vi "Configure Trigger (Setup and Hold).vi"(5 "Slope Type (0: Positive)":i32(ring) items=["Positive", "Negative"], 6 "Setup Time (3E-9 S)":dbl=3e-09, 7 "Hold Time (2E-9 S)":dbl=2e-09, 8 "error in (no error)":errorcluster, 9 "Data Source (1: Channel 2)":i32(ring)=1 items=["Channel 1"=0, "Channel 2"=1, "Channel 3"=2, "Channel 4"=3, "D0"=13, "D1"=14, "D2"=15, "D3"=16, "D4"=17, "D5"=18, "D6"=19, "D7"=20, "D8"=21, "D9"=22, "D10"=23, "D11"=24, "D12"=25, "D13"=26, "D14"=27, "D15"=28, "External"=29], 10 "Clock Source (0: Channel 1)":i32(ring) items=["Channel 1"=0, "Channel 2"=1, "Channel 3"=2, "Channel 4"=3, "D0"=13, "D1"=14, "D2"=15, "D3"=16, "D4"=17, "D5"=18, "D6"=19, "D7"=20, "D8"=21, "D9"=22, "D10"=23, "D11"=24, "D12"=25, "D13"=26, "D14"=27, "D15"=28, "External"=29], 11 "VISA resource name":refnum<visa-resource-name>) -> (0 "error out":errorcluster, 3 "VISA resource name out":refnum<visa-resource-name>)   [LabVIEW 2016, in "Agilent 2000 3000 X-Series.lvlib"]
doc: "Configures the setup and hold trigger mode."
uses:
  Agilent 2000 3000 X-Series.lvlib
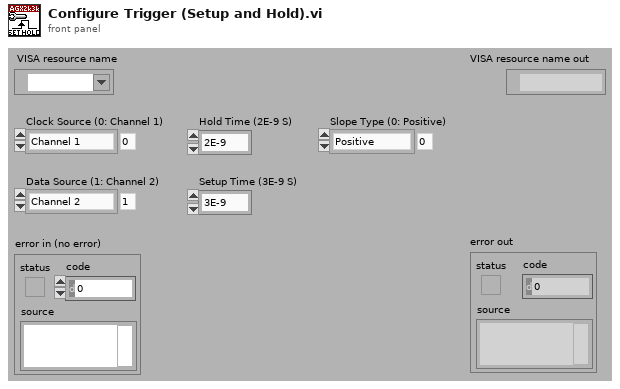
[diagram p1: front panel]
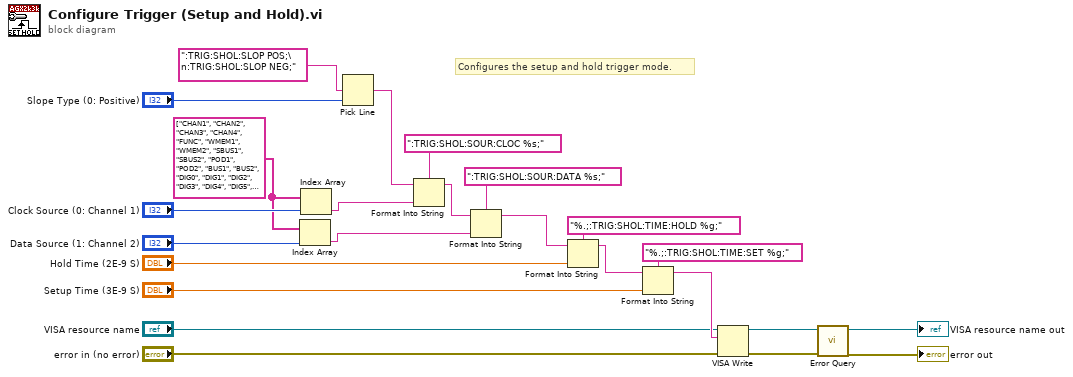
[diagram p0: block diagram]
diagram:
  w3 = string[] ["CHAN1", "CHAN2", "CHAN3", "CHAN4", "FUNC", "WMEM1", "WMEM2", "SBUS1", "SBUS2", "POD1", "POD2", "BUS1", "BUS2", "DIG0", "DIG1", "DIG2", "DIG3", "DIG4", "DIG5", "DIG6", "DIG7", "DIG8", "DIG9", "DIG10", "DIG11", "DIG12", "DIG13", "DIG14", "DIG15", "EXT", "LINE", "WGEN"]
  # "Configures the setup and hold trigger mode."
  n1 = Index Array(array=w3, index="Data Source (1: Channel 2)") -> (element=w2:string)
  n2 = Index Array(array=w3, index="Clock Source (0: Channel 1)") -> (element=w4:string)
  n3 = Pick Line(multi-line string=":TRIG:SHOL:SLOP POS;\n:TRIG:SHOL:SLOP NEG;", line index="Slope Type (0: Positive)") -> (output string=w9:string)  [unwired: 1 out]
  n4 = Format Into String(format string=":TRIG:SHOL:SOUR:CLOC %s;", initial string=w9, w4) -> (resulting string=w7:string)  [unwired: 1 in, 1 out]
  n5 = Format Into String(format string=":TRIG:SHOL:SOUR:DATA %s;", initial string=w7, w2) -> (resulting string=w8:string)  [unwired: 1 in, 1 out]
  n6 = Format Into String(format string="%.;:TRIG:SHOL:TIME:HOLD %g;", initial string=w8, "Hold Time (2E-9 S)") -> (resulting string=w20:string)  [unwired: 1 in, 1 out]
  n7 = Format Into String(format string="%.;:TRIG:SHOL:TIME:SET %g;", initial string=w20, "Setup Time (3E-9 S)") -> (resulting string=w17:string)  [unwired: 1 in, 1 out]
  n8 = VISA Write(VISA resource name="VISA resource name", write buffer=w17, error in (no error)="error in (no error)") -> (VISA resource name out=w14:refnum<visa-resource-name>, error out=w13:errorcluster)  [unwired: 1 out]
  n9 = call "Error Query.vi"("error in (no error)"=w13, "VISA resource name"=w14) -> ("error out"=→"error out":errorcluster, "VISA resource name out"=→"VISA resource name out":refnum<visa-resource-name>)  [unwired: 8 out]
